vi "set_outlets.vi"(8 "Switch status":bool[](array[boolean])=[FALSE, FALSE, FALSE, FALSE, FALSE, FALSE, FALSE, FALSE], 11 "IP / Hostname":string="172.20.125.112") -> ()   [LabVIEW 2017]
panel:
  out "Returns":string[](array[string])
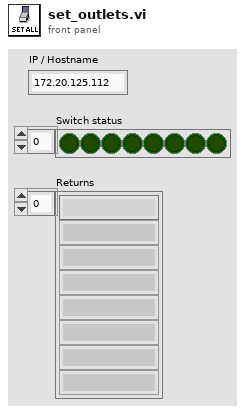
[diagram p1: front panel]
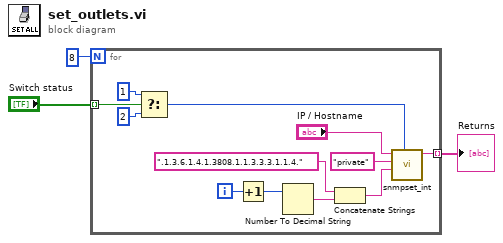
[diagram p0: block diagram]
diagram:
  n1 = for {
    N: 8 -> [_]
    tunnel: "Switch status" -> [w7] mode=indexing
    tunnel: [w8] -> w1 mode=indexing
    i -> [w13]
    n2 = Select(t=1, s=w7, f=2) -> (s? t:f=w4:i32)
    n3 = Increment(x=w13) -> (x+1=w12:i32)
    n4 = Number To Decimal String(number=w12) -> (decimal integer string=w10:string)  [unwired: 1 in]
    n5 = Concatenate Strings(".1.3.6.1.4.1.3808.1.1.3.3.3.1.1.4." ("OID"), w10) -> (w9:string)
    n6 = call "snmpset_int.vi"("value"=w4, "OID"=w9, "community"="private", "IP / Hostname"="IP / Hostname") -> ("return"=w8:string)  [unwired: 6 in, 1 out]
  }
  "Returns" <- w1
